vi "Reinitialize All To Default Method-placeContent.vi"   [LabVIEW 2017]
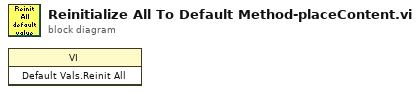
[diagram p0: block diagram]
diagram:
  n1 = invoke class="VI" method="Default Vals.Reinit All"() -> ()  [unwired: 3 in, 3 out]
